vi "Init.vi"(0 "ClassWriter in":refnum<class "ClassWriter.lvclass">, 1 "UseProgressWindow(true)":bool=TRUE, 5 "error in (no error)":errorcluster, 7 "ClassFileMayBeReadOnly(False)":bool, 8 "LVClassLibrary Refnum":refnum<vi>) -> (14 "ClassWriter out":refnum<class "ClassWriter.lvclass">, 19 "error out":errorcluster)   [LabVIEW 2020, in "ClassWriter.lvclass"]
uses:
  <resource>/Framework/Providers/Open_GDS/ClassProviders/Provider_BaseClassInterface/ClassWriter_class/ClassWriter.lvclass
  <resource>/Framework/Providers/Open_GDS/ClassProviders/Provider_BaseClassInterface/ClassWriter_class/ClassWriter.lvclass/ClassWriter.ctl
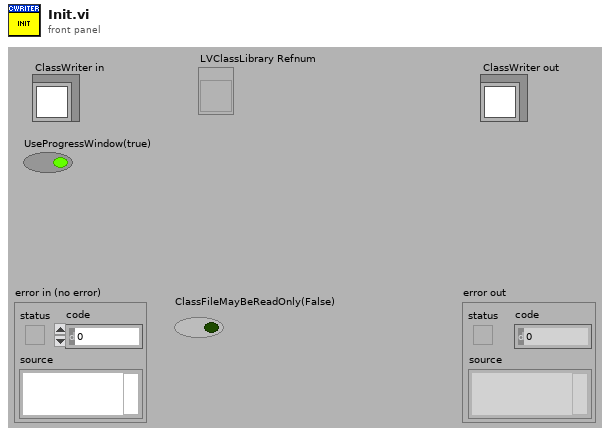
[diagram p1: front panel]
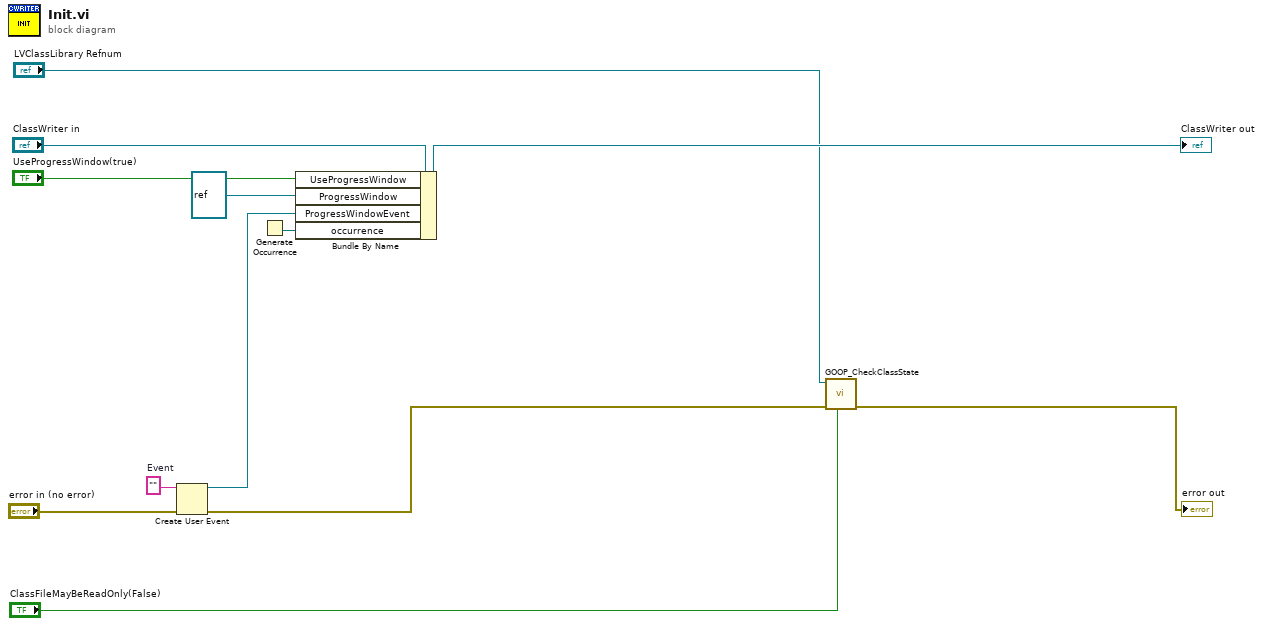
[diagram p0: block diagram]
diagram:
  w8 = ""  # Event
  n1 = Create User Event(user event datatype=w8, error in="error in (no error)") -> (user event=w6:refnum<user-event>, error out=w3:errorcluster)
  n2 = Generate Occurrence() -> (w7:refnum<k4>)
  n3 = Bundle By Name(cluster="ClassWriter in", "UseProgressWindow"="UseProgressWindow(true)", "ProgressWindow"=refnum<vi> refnum ("PregressWindow"), "ProgressWindowEvent"=w6, "occurrence"=w7) -> (→"ClassWriter out":refnum<class "ClassWriter.lvclass">)
  n4 = call <resource>:"GOOP_CheckClassState.vi"("ClassFileMayBeReadOnly(False)"="ClassFileMayBeReadOnly(False)", "error in"=w3, "Library Refnum"="LVClassLibrary Refnum") -> ("error out"=→"error out":errorcluster)  [unwired: 8 in]
